vi "TdmsPropertiesToVariantAttributes.vi"(9 "Tdms Properties":T1[](array[typedef]), 11 "Variant in":variant) -> (3 "Variant out":variant)   [LabVIEW 2017, in "Tdms.lvlib"]
uses:
  <vilib>/addons/InsightCM/Utilities/Tdms/Tdms.lvlib
  <vilib>/addons/InsightCM/Utilities/Tdms/controls/Property.ctl
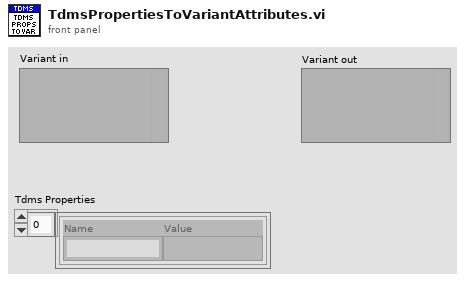
[diagram p1: front panel]
types:
  T1 = typedef "Tdms.lvlib/Property.ctl" = cluster{"Name":string, "Value":variant}
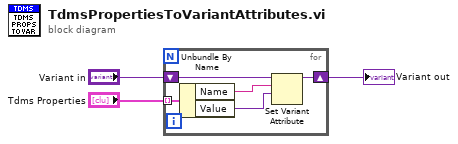
[diagram p0: block diagram]
diagram:
  n1 = for {
    shift-right: [w8] -> w3
    shift-left: "Variant in" -> [w7]
    tunnel: "Tdms Properties" -> [w6] mode=indexing
    n2 = Unbundle By Name(w6) -> ("Name"=w5:string, "Value"=w4:variant)
    n3 = Set Variant Attribute(Variant=w7, name=w5, value=w4) -> (Variant out=w8:variant)  [unwired: 1 in, 2 out]
  }
  "Variant out" <- w3
